vi "OAT Order Grids for Frequency-RPM Plot.vi"(6 "order grids":cluster{"start":dbl, "multiplier":dbl}={"start"=1.0, "multiplier"=1.0} {"multiplier" format="%.2f"; "start" format="%.2f"}, 7 "intensity graph ref":refnum<vi>, 8 "error in (no error)":errorcluster, 9 "unit labels":T1={"X unit"="RPM", "Y unit"="Hz", "Z unit"="dB ref 1.0E+0 g"}, 10 "scales":T2 {"Y scale"."multiplier" format="%.2f"; "Y scale"."offset" format="%.2f"; "X scale"."multiplier" format="%.2f"; "X scale"."offset" format="%.2f"}, 11 "F-RPM map":dbl[][](array[numeric]) format="%.2f") -> (0 "error out":errorcluster, 1 "Z unit":string, 3 "intensity graph value":dbl[][](array[numeric]) format="%.2f")   [LabVIEW 2017]
doc: "Draws order grids on a frequency-rpm spectral map."
uses:
  <vilib>/Analysis/NI_AALBase.lvlib
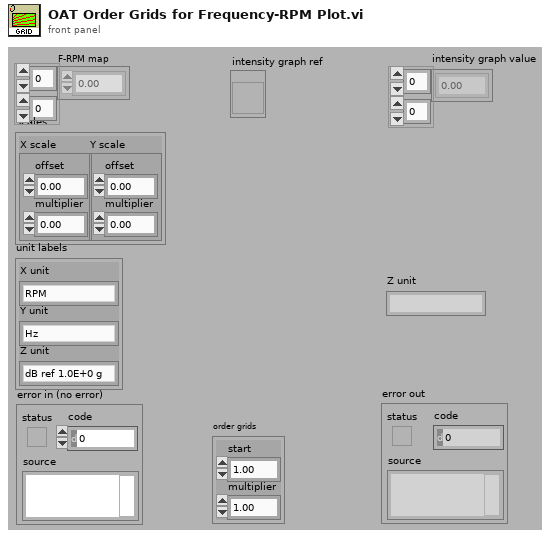
[diagram p1: front panel]
types:
  T1 = cluster{"X unit":string, "Y unit":string, "Z unit":string}
  T2 = cluster{"X scale":cluster{"offset":dbl, "multiplier":dbl}, "Y scale":cluster{"offset":dbl, "multiplier":dbl}}
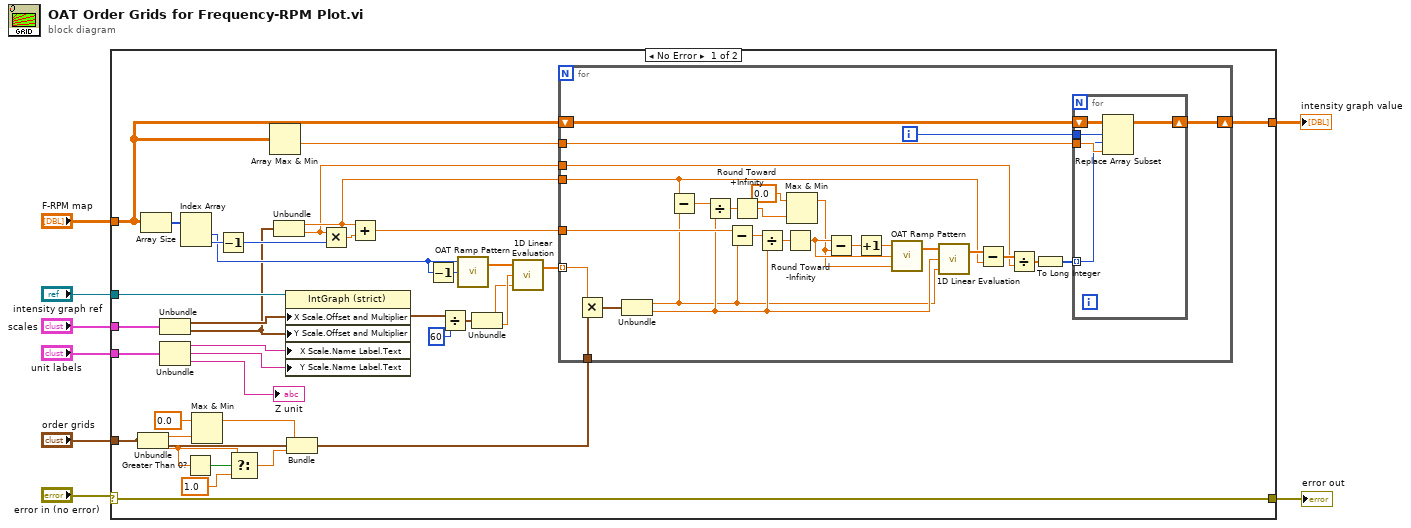
[diagram p0: block diagram]
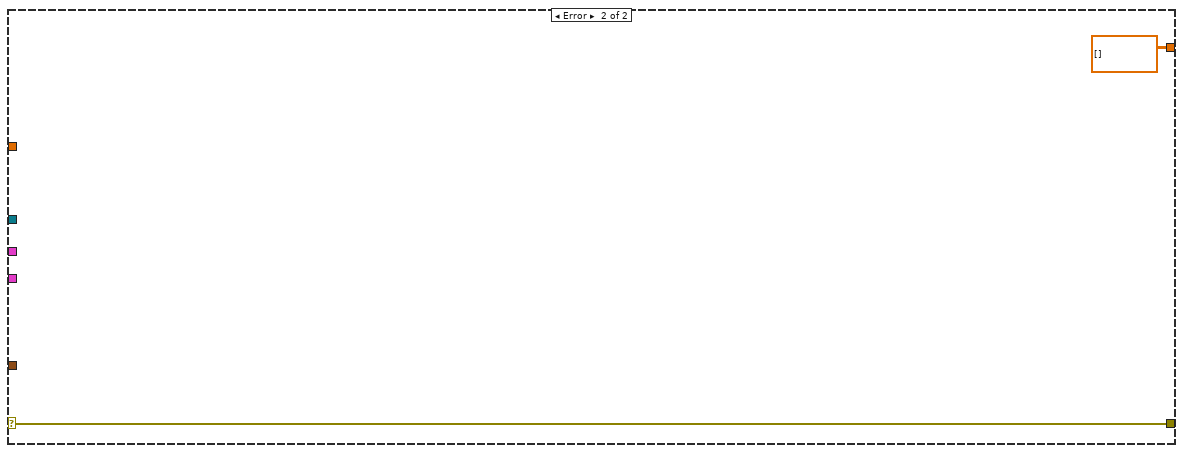
[diagram p2: hidden frame]
diagram:
  n1 = case shown="No Error" "error in (no error)" {
    selector: "error in (no error)" -> [w9 w78]
    tunnel: "scales" -> [w42 _]
    tunnel: "unit labels" -> [w41 _]
    tunnel: "intensity graph ref" -> [w31 _]
    tunnel: "F-RPM map" -> [w30 _]
    tunnel: [w29 dbl[][] [] ("F-RPM map")] -> w4
    tunnel: "order grids" -> [w11 _]
    tunnel: [w9 w78] -> w1
    frame No Error {
      n2 = Unbundle(w11) -> ("start"=w18:dbl, "multiplier"=w15:dbl)
      n3 = Array Size(array=w30) -> (size(s)=w39:i32[])
      n4 = Unbundle(w42) -> ("X scale"=w28:cluster{"offset":dbl, "multiplier":dbl}, "Y scale"=w20:cluster{"offset":dbl, "multiplier":dbl})
      n5 = Unbundle(w41) -> ("X unit"=w44:string, "Y unit"=w43:string, "Z unit"=→"Z unit":string)
      n6 = Index Array(array=w39) -> (element #1=w26:i32, element #2=w38:i32)  [unwired: 2 in]
      n7 = Greater Than 0?(x=w15) -> (x > 0?=w16:bool)
      n8 = Max & Min(x=0.0, y=w18) -> (max(x,y)=w12:dbl)  [unwired: 1 out]
      n9 = Decrement(x=w38) -> (x-1=w36:i32)
      n10 = Select(t=w15, s=w16, f=1.0) -> (s? t:f=w13:dbl)
      n11 = Array Max & Min(array=w30) -> (min value=w32:dbl)  [unwired: 3 out]
      n12 = Unbundle(w20) -> ("offset"=w35:dbl, "multiplier"=w33:dbl)
      n13 = property on="Property Node" class="IntGraph (strict)"(reference=w31, "X Scale.Offset and Multiplier"=w28, "Y Scale.Offset and Multiplier"=w20, "X Scale.Name Label.Text"=w44, "Y Scale.Name Label.Text"=w43) -> ()  [unwired: 1 in, 2 out]
      n14 = Bundle(cluster=w11, "start"=w12, "multiplier"=w13) -> (w10:cluster{"start":dbl, "multiplier":dbl})
      n15 = Multiply(x=w33, y=w36) -> (x*y=w37:dbl)
      n16 = Add(x=w35, y=w37) -> (x+y=w34:dbl)
      n17 = Decrement(x=w26) -> (x-1=w25:i32)
      n18 = Divide(x=w28, y=60) -> (x/y=w23:cluster{"offset":dbl, "multiplier":dbl})
      n19 = call <vilib>:"OAT Ramp Pattern.vi"("end"=w25, "samples"=w26) -> ("Ramp Pattern"=w24:dbl[])  [unwired: 1 in, 1 out]
      n20 = Unbundle(w23) -> ("offset"=w21:dbl, "multiplier"=w22:dbl)
      n21 = call <vilib>:"1D Linear Evaluation.vi"("offset"=w21, "scale"=w22, "X"=w24) -> ("Y[i]=X[i]*a+b"=w19:dbl[])  [unwired: 1 out]
      n22 = for {
        tunnel: w35 -> [w62]
        tunnel: w34 -> [w67]
        tunnel: w33 -> [w60]
        tunnel: w32 -> [w52]
        shift-right: [w48] -> w29
        shift-left: w30 -> [w49]
        tunnel: w19 -> [w46] mode=indexing
        tunnel: w10 -> [w45]
        i -> [w47]
        n23 = Multiply(x=w46, y=w45) -> (x*y=w71:cluster{"start":dbl, "multiplier":dbl})
        n24 = Unbundle(w71) -> ("start"=w64:dbl, "multiplier"=w65:dbl)
        n25 = Subtract(x=w62, y=w64) -> (x-y=w70:dbl)
        n26 = Divide(x=w70, y=w65) -> (x/y=w69:dbl)
        n27 = Subtract(x=w67, y=w64) -> (x-y=w68:dbl)
        n28 = Round Toward +Infinity(x=w69) -> (ceil(x): smallest int >= x=w55:dbl)
        n29 = Divide(x=w68, y=w65) -> (x/y=w66:dbl)
        n30 = Round Toward -Infinity(1:w66) -> (0:w56:dbl)
        n31 = Max & Min(x=0.0, y=w55) -> (max(x,y)=w50:dbl)  [unwired: 1 out]
        n32 = Subtract(x=w56, y=w50) -> (x-y=w58:dbl)
        n33 = Increment(x=w58) -> (x+1=w57:dbl)
        n34 = call <vilib>:"OAT Ramp Pattern.vi"("start"=w50, "end"=w56, "samples"=w57) -> ("Ramp Pattern"=w54:dbl[])  [unwired: 1 out]
        n35 = call <vilib>:"1D Linear Evaluation.vi"("offset"=w64, "scale"=w65, "X"=w54) -> ("Y[i]=X[i]*a+b"=w63:dbl[])  [unwired: 1 out]
        n36 = Subtract(x=w63, y=w62) -> (x-y=w61:dbl[])
        n37 = Divide(x=w61, y=w60) -> (x/y=w59:dbl[])
        n38 = To Long Integer(number=w59) -> (32bit integer=w53:i32[])
        n39 = for {
          shift-right: [w75] -> w48
          shift-left: w49 -> [w76]
          tunnel: w53 -> [w73] mode=indexing
          tunnel: w52 -> [w74]
          tunnel: w47 -> [w72]
          n40 = Replace Array Subset(array=w76, new element=w74, index (row)=w72, index (col)=w73) -> (w75:dbl[][])
        }
      }
    }
    frame Error {
    }
  }
  "intensity graph value" <- w4
  "error out" <- w1
